vi "IMAQ FPGA Skip Image Transfer to Host.vi"(7 "Reset":bool, 8 "Output Valid In":bool, 10 "Image Skip Count":u16, 11 "EOI In":bool) -> (0 "Output Valid Out":bool, 3 "Number of Frames Transferred":u64)   [LabVIEW 2020, in "NI_VDM_FPGA_Basics.lvlib"]
uses:
  <vilib>/visionFPGA/NI_VDM_FPGA_Basics.lvlib
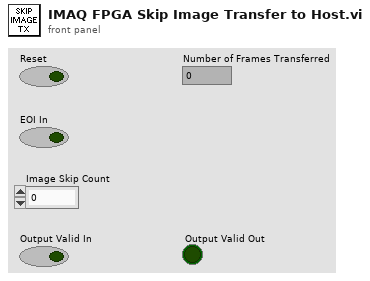
[diagram p1: front panel]
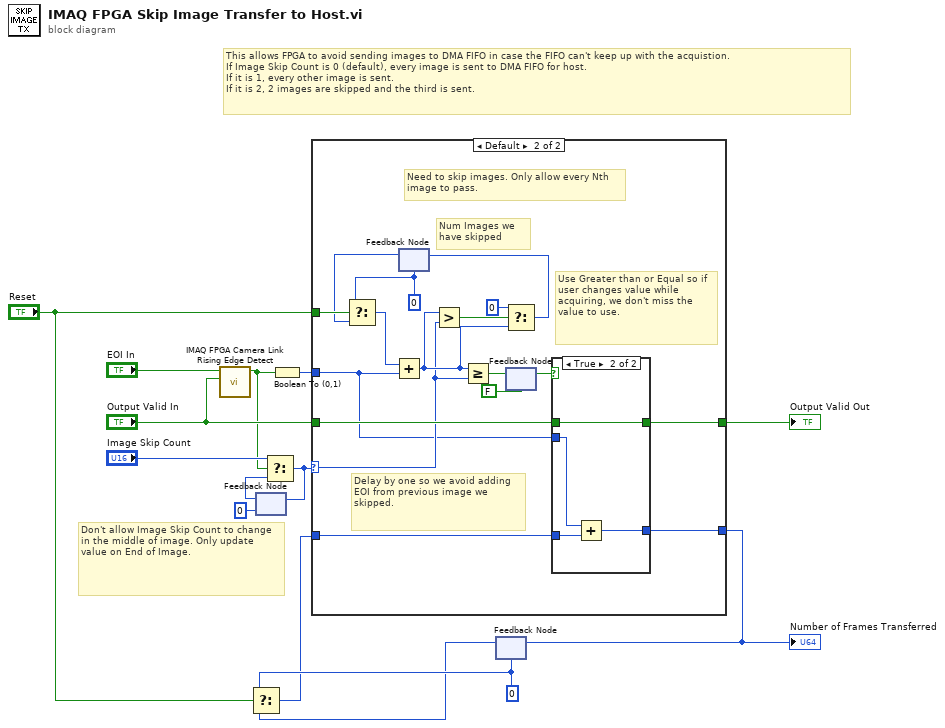
[diagram p0: block diagram]
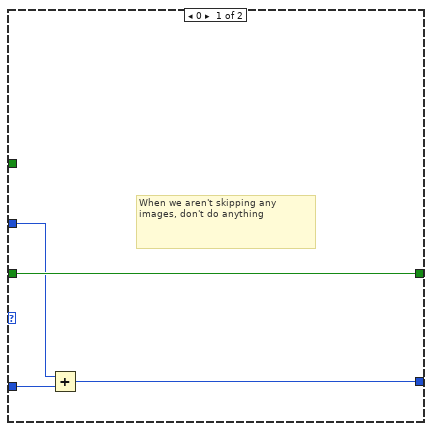
[diagram p2: hidden frame]
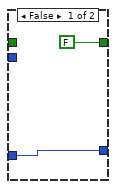
[diagram p3: hidden frame]
diagram:
  w3 = u64 0 ("Image Skip Count")
  # "Don't allow Image Skip Count to change in the middle of image. Only update value on End of Image."
  # "This allows FPGA to avoid sending images to DMA FIFO in case the FIFO can't keep up with the acquistion. \nIf Image Skip Count is 0 (default), every image is sent to DMA FIFO for host. \nIf it is 1, every other image is sent.\nIf it is 2, 2 images are skipped and the third is sent."
  n1 = call <vilib>:"IMAQ FPGA Camera Link Rising Edge Detect.vi"("Input Valid"="Output Valid In", "Input"="EOI In") -> ("Rising Edge"=w7:bool)  [unwired: 9 in]
  n2 = feedback #1(u16 0 ("Image Skip Count")) -> (w10:u16)
  n3 = Select(t="Image Skip Count", s=w7, f=w10) -> (s? t:f=w9:u16)
  n4 = feedback-in #1(w9) -> ()
  n5 = Boolean To (0,1)(Boolean=w7) -> (0, 1=w6:i16)
  n6 = feedback #2(w3) -> (w1:u64)
  n7 = Select(t=w3, s="Reset", f=w1) -> (s? t:f=w2:u64)
  n8 = case shown="Default" w9 {
    selector: w9 -> [_ w27]
    tunnel: "Output Valid In" -> [w18 w33]
    tunnel: [w18 w26] -> w14
    tunnel: w6 -> [w16 w24]
    tunnel: w2 -> [w17 w25]
    tunnel: [w15 w23] -> w5
    tunnel: "Reset" -> [_ w22]
    frame 0 {
      # "When we aren't skipping any images, don't do anything"
      n9 = Add(x=w16, y=w17) -> (x+y=w15:u64)
    }
    frame Default {
      w19 = u16 0
      # "Delay by one so we avoid adding EOI from previous image we skipped."
      # "Need to skip images. Only allow every Nth image to pass."
      # "Num Images we have skipped"
      # "Use Greater than or Equal so if user changes value while acquiring, we don't miss the value to use."
      n10 = feedback #3(w19) -> (w21:u16)
      n11 = Select(t=w19, s=w22, f=w21) -> (s? t:f=w20:u16)
      n12 = Add(x=w20, y=w24) -> (x+y=w29:u16)
      n13 = Greater?(x=w29, y=w27) -> (0:w28:bool)
      n14 = Greater Or Equal?(x=w29, y=w27) -> (x >= y?=w32:bool)
      n15 = Select(t=u16 0, s=w28, f=w29) -> (s? t:f=w34:u16)
      n16 = feedback-in #3(w34) -> ()
      n17 = feedback #4(FALSE) -> (w31:bool)
      n18 = feedback-in #4(w32) -> ()
      n19 = case shown="True" w31 {
        tunnel: w33 -> [_ w41]
        tunnel: [FALSE ("Output Valid in") w41] -> w26
        tunnel: w25 -> [w36 w40]
        tunnel: w24 -> [_ w39]
        tunnel: [w36 w38] -> w23
        frame False {
        }
        frame True {
          n20 = Add(x=w39, y=w40) -> (x+y=w38:u64)
        }
      }
    }
  }
  "Output Valid Out" <- w14
  "Number of Frames Transferred" <- w5
  n21 = feedback-in #2(w5) -> ()
